vi "TEST - Get Header from TD.vi"(8 "error in (no error)":errorcluster) -> (0 "error out":errorcluster, 2 "pass":bool)   [LabVIEW 2020, in "test_openg_variant.lvlib"]
uses:
  test_openg_variant.lvlib
  source/library/Type Descriptor.ctl
  source/library/Type Descriptor Header.ctl
  source/library/Type Descriptor Enumeration.ctl
  <vilib>/addons/_JKI Toolkits/Caraya/classes/Assert/Assert True.vi
  source/library/openg_variant.lvlib
  <vilib>/addons/_JKI Toolkits/Caraya/classes/Test/Test.lvclass
  <vilib>/addons/_JKI Toolkits/Caraya/classes/Assert/Assert.lvclass
panel:
  out "Test Name":string
  out "Failures":T4(array[cluster]) {"result"."Type Descriptor Header"."type" format="%.0x"; "exected result"."Type Descriptor Header"."type" format="%.0x"}
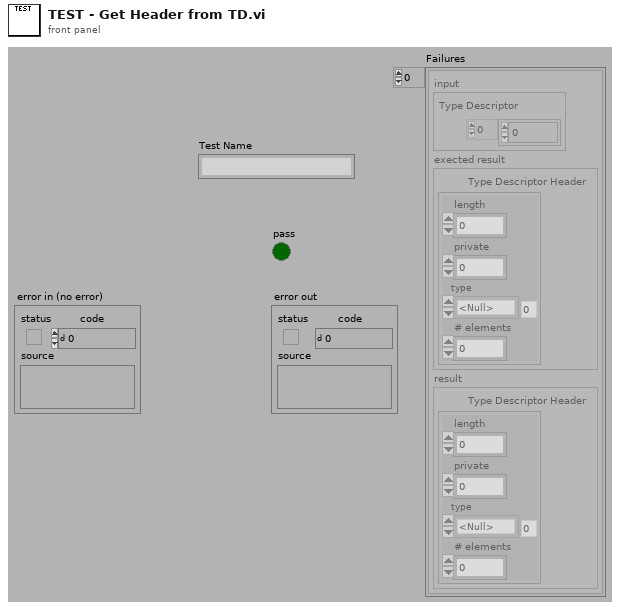
[diagram p1: front panel]
types:
  T1 = typedef "openg_variant.lvlib/Type Descriptor.ctl" = i16[]
  T2 = typedef "openg_variant.lvlib/Type Descriptor Header.ctl" = cluster{"length":u16, "private":u8, "type":T3, "# elements":u16}
  T3 = typedef "openg_variant.lvlib/Type Descriptor Enumeration.ctl" = enum8{"<Null>", "I8", "I16", "I32", "I64", "U8", "U16", "U32", "U64", "SGL", "DBL", "EXT", "CSG", "CDB", "CXT", "0x0F", "0x10", "0x11", "0x12", "0x13", "0x14", "Enum U8", "Enum U16", "Enum U32", "Enum U64", "SGL PQ", "DBL PQ", "EXT PQ", "CSG PQ", "CDB PQ", "CXT PQ", "0x1F", "0x20", "Boolean", "0x22", "0x23", "0x24", "0x25", "0x26", "0x27", "0x28", "0x29", "0x2A", "0x2B", "0x2C", "0x2D", "0x2E", "0x2F", "String", "0x31", "Path", "Pict", "0x34", "0x35", "0x36", "DAQ", "0x38", "0x39", "0x3A", "0x3B", "0x3C", "0x3D", "0x3E", "0x3F", "Array", "0x41", "0x42", "0x43", "0x44", "0x45", "0x46", "0x47", "0x48", "0x49", "0x4A", "0x4B", "0x4C", "0x4D", "0x4E", "0x4F", "Cluster", "0x51", "0x52", "Variant", "Waveform", "0x55", "0x56", "0x57", "0x58", "0x59", "0x5A", "0x5B", "0x5C", "0x5D", "0x5E", "Fixed Point", "0x60", "0x61", "0x62", "0x63", "0x64", "0x65", "0x66", "0x67", "0x68", "0x69", "0x6A", "0x6B", "0x6C", "0x6D", "0x6E", "0x6F", "Refnum", "0x71", "0x72", "Set Collection", "Map Collection"}
  T4 = cluster{"input":cluster{"Type Descriptor":T1}, "exected result":cluster{"Type Descriptor Header":T2}, "result":cluster{"Type Descriptor Header":T2}}[]
  T5 = cluster{"input":cluster{"Type Descriptor":T1}, "exected result":cluster{"Type Descriptor Header":T2}, "result":cluster{"Type Descriptor Header":T2}}
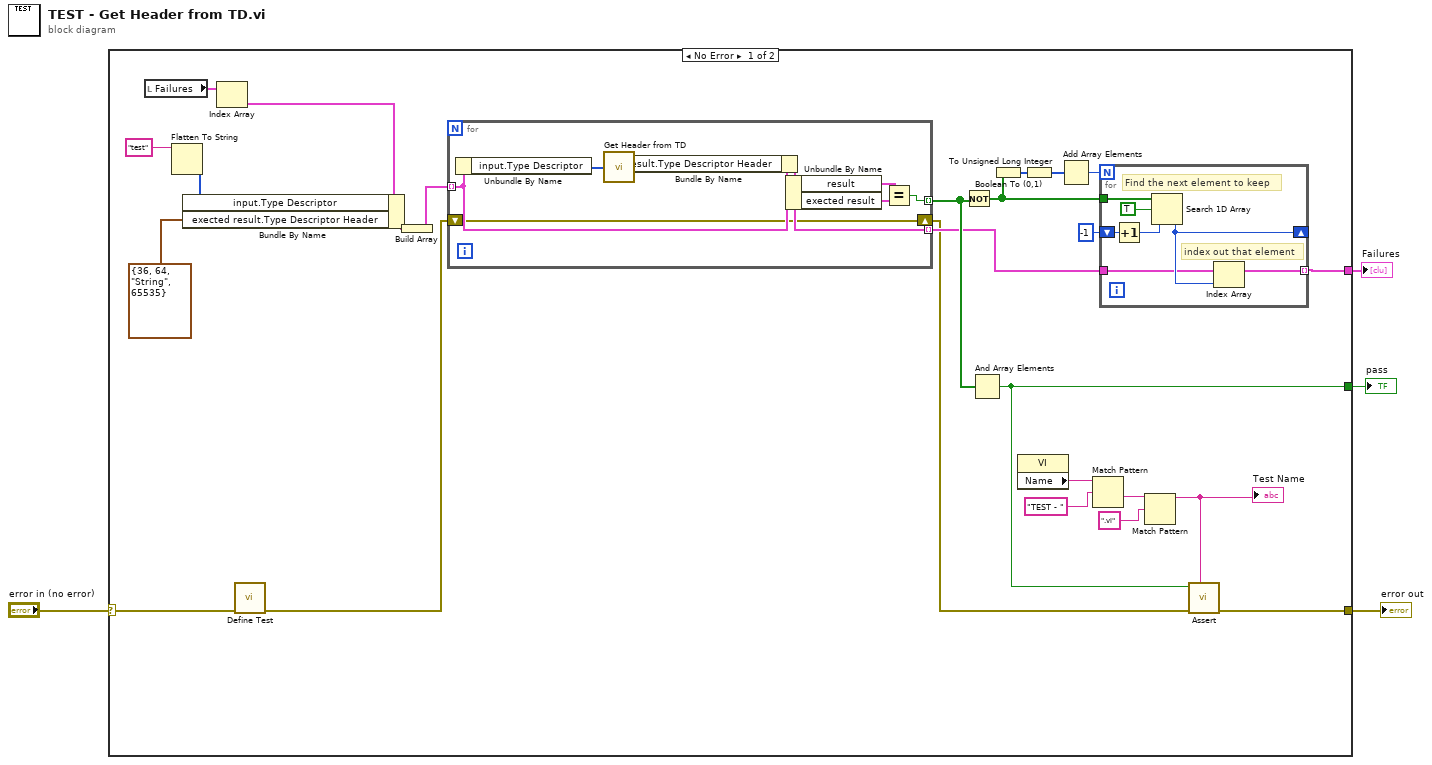
[diagram p0: block diagram]
diagram:
  n1 = case shown="No Error" "error in (no error)" {
    selector: "error in (no error)" -> [w6 w45]
    tunnel: [w7 _] -> w4
    tunnel: [w9 w45] -> w2
    tunnel: [w22 _] -> w1
    frame No Error {
      n2 = local read "Failures"() -> (w19:T4)
      n3 = Flatten To String(anything="test" ("exected result.Object Type")) -> (type string=w17:i16[])  [unwired: 3 in, 2 out]
      n4 = Index Array(array=w19) -> (element=w18:T5)  [unwired: 1 in]
      n5 = Bundle By Name(cluster=w18, "input.Type Descriptor"=w17, "exected result.Type Descriptor Header"=T2 {"length"=36, "private"=64, "type"=enum."String", "# elements"=65535} ("Type Descriptor Header")) -> (w21:T5)
      n6 = call <vilib>:"Define Test.vi"("error in (no error)"=w6) -> ("error out"=w5:errorcluster)  [unwired: 9 in, 1 out]
      n7 = Build Array(w21) -> (w20:T4)
      n8 = for {
        tunnel: w20 -> [w43] mode=indexing
        tunnel: [w44] -> w24 mode=indexing
        tunnel: [w42] -> w23 mode=indexing
        shift-right: [w37] -> w8
        shift-left: w5 -> [w37]
        n9 = Unbundle By Name(w43) -> ("input.Type Descriptor"=w39:T1)
        n10 = call "Get Header from TD.vi"("Type Descriptor"=w39) -> ("Type Descriptor Header"=w38:T2)
        n11 = Bundle By Name(cluster=w43, "result.Type Descriptor Header"=w38) -> (w42:T5)
        n12 = Unbundle By Name(w42) -> ("result"=w41:cluster{"Type Descriptor Header":T2}, "exected result"=w40:cluster{"Type Descriptor Header":T2})
        n13 = Equal?(x=w41, y=w40) -> (x = y?=w44:bool)
      }
      n14 = Not(x=w24) -> (.not. x?=w26:bool[])
      n15 = And Array Elements(Boolean array=w24) -> (logical AND=w7:bool)
      n16 = Boolean To (0,1)(Boolean=w26) -> (0, 1=w27:i16[])
      n17 = property class="VI"() -> ("Name"=w13:string)  [unwired: 2 in, 2 out]
      n18 = To Unsigned Long Integer(number=w27) -> (unsigned 32bit integer=w25:u32[])
      n19 = Add Array Elements(numeric array=w25) -> (sum=w28:u32)
      n20 = Match Pattern(string=w13, regular expression="TEST - ") -> (after substring=w14:string)  [unwired: 1 in, 3 out]
      n21 = for {
        N: w28 -> [_]
        tunnel: w23 -> [w32]
        tunnel: w26 -> [w36]
        shift-right: [w33] -> _
        shift-left: -1 ("start index (0)") -> [w34]
        tunnel: [w31] -> w22 mode=indexing
        # "index out that element"
        # "Find the next element to keep"
        n22 = Increment(x=w34) -> (x+1=w30:i32)
        n23 = Search 1D Array(1D array=w36, element=TRUE, start index (0)=w30) -> (index of element=w33:i32)
        n24 = Index Array(array=w32, index=w33) -> (element=w31:T5)
      }
      n25 = Match Pattern(string=w14, regular expression=".vi") -> (before substring=w10:string)  [unwired: 1 in, 3 out]
      "Test Name" <- w10
      n26 = call-poly <vilib>:"Assert.vi"("Label"=w10, "error in (no error)"=w8, "True?"=w7) -> ("error out"=w9:errorcluster)  [unwired: 7 in, 1 out]
    }
    frame Error {
    }
  }
  "pass" <- w4
  "error out" <- w2
  "Failures" <- w1
